vi "MGCC_FntStaMach_Control panel loop.vi"   [LabVIEW 2016]
doc: "This VI is used to convert the flags into events."
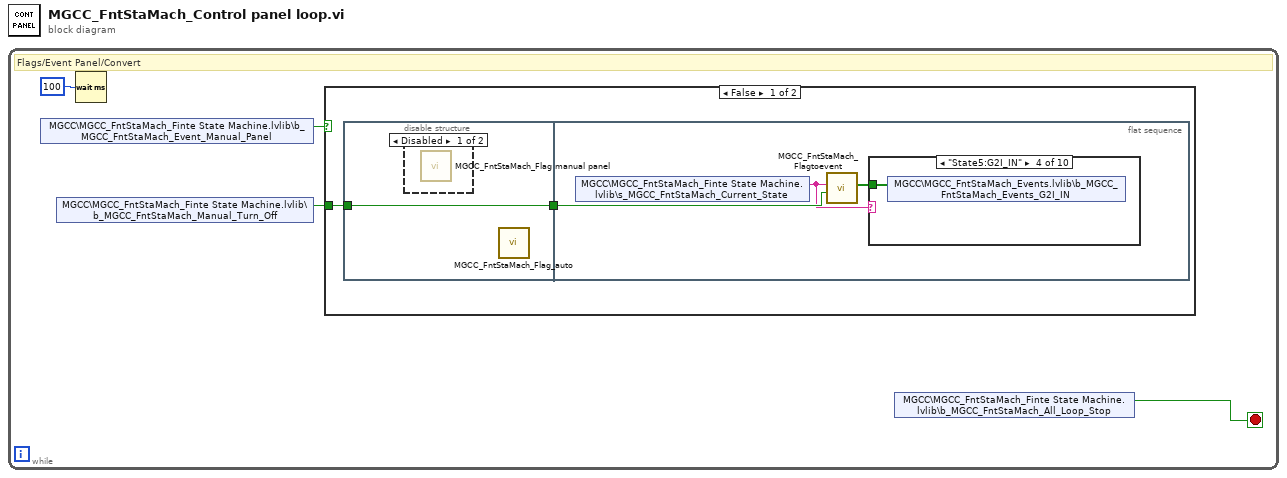
[diagram p0: block diagram]
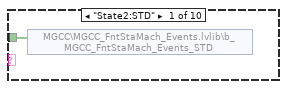
[diagram p3: hidden frame]
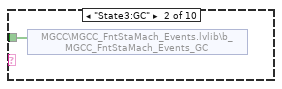
[diagram p4: hidden frame]
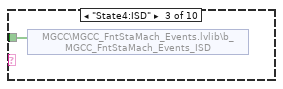
[diagram p5: hidden frame]
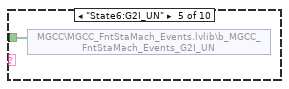
[diagram p6: hidden frame]
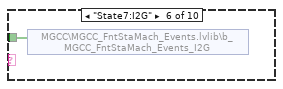
[diagram p7: hidden frame]
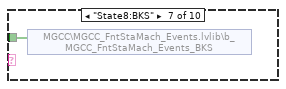
[diagram p8: hidden frame]
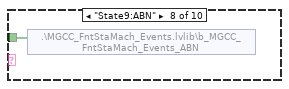
[diagram p9: hidden frame]
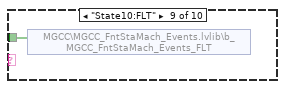
[diagram p10: hidden frame]
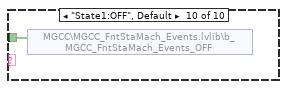
[diagram p11: hidden frame]
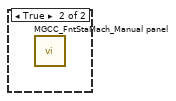
[diagram p12: hidden frame]
diagram:
  n1 = while {
    stop <- w3 stop-if-true
    # "Flags/Event Panel/Convert"
    n2 = shared-variable "MGCC\\MGCC_FntStaMach_Finte State Machine.lvlib\\b_MGCC_FntStaMach_Event_Manual_Panel"() -> (w2:bool)  [unwired: 1 in, 1 out]
    n3 = shared-variable "MGCC\\MGCC_FntStaMach_Finte State Machine.lvlib\\b_MGCC_FntStaMach_Manual_Turn_Off"() -> (w1:bool)  [unwired: 1 in, 1 out]
    n4 = Wait (ms)(milliseconds to wait=u32 100) -> ()  [unwired: 1 out]
    n5 = case shown="False" w2 {
      tunnel: w1 -> [w6 _]
      frame False {
        n6 = flat-sequence {
          tunnel: w6 -> [w7]
          tunnel: [w7] -> w5
          tunnel: w5 -> [w10]
          frame #0 {
            n7 = disable-structure shown="Disabled" {
              frame Disabled {
                n8 = call "MGCC_FntStaMach_Flag manual panel.vi"() -> ()  [unwired: 12 in]
              }
              frame Enabled {
              }
            }
            n9 = call "MGCC_FntStaMach_Flag_auto.vi"() -> ()  [unwired: 1 out]
          }
          frame #1 {
            n10 = shared-variable "MGCC\\MGCC_FntStaMach_Finte State Machine.lvlib\\s_MGCC_FntStaMach_Current_State"() -> (w8:string)  [unwired: 1 in, 1 out]
            n11 = call "MGCC_FntStaMach_Flagtoevent.vi"("M_OFF"=w10, "Pre_state"=w8) -> ("Event"=w9:bool[])  [unwired: 8 in, 1 out]
            n12 = case shown="\"State5:G2I_IN\"" w8 {
              tunnel: w9 -> [w11 w12 w13 w14 w15 w16 w17 w18 w19 w20]
              frame "State2:STD" {
                n13 = shared-variable "MGCC\\MGCC_FntStaMach_Events.lvlib\\b_MGCC_FntStaMach_Events_STD"(w11) -> ()  [unwired: 1 in, 1 out]
              }
              frame "State3:GC" {
                n14 = shared-variable "MGCC\\MGCC_FntStaMach_Events.lvlib\\b_MGCC_FntStaMach_Events_GC"(w12) -> ()  [unwired: 1 in, 1 out]
              }
              frame "State4:ISD" {
                n15 = shared-variable "MGCC\\MGCC_FntStaMach_Events.lvlib\\b_MGCC_FntStaMach_Events_ISD"(w13) -> ()  [unwired: 1 in, 1 out]
              }
              frame "State5:G2I_IN" {
                n16 = shared-variable "MGCC\\MGCC_FntStaMach_Events.lvlib\\b_MGCC_FntStaMach_Events_G2I_IN"(w14) -> ()  [unwired: 1 in, 1 out]
              }
              frame "State6:G2I_UN" {
                n17 = shared-variable "MGCC\\MGCC_FntStaMach_Events.lvlib\\b_MGCC_FntStaMach_Events_G2I_UN"(w15) -> ()  [unwired: 1 in, 1 out]
              }
              frame "State7:I2G" {
                n18 = shared-variable "MGCC\\MGCC_FntStaMach_Events.lvlib\\b_MGCC_FntStaMach_Events_I2G"(w16) -> ()  [unwired: 1 in, 1 out]
              }
              frame "State8:BKS" {
                n19 = shared-variable "MGCC\\MGCC_FntStaMach_Events.lvlib\\b_MGCC_FntStaMach_Events_BKS"(w17) -> ()  [unwired: 1 in, 1 out]
              }
              frame "State9:ABN" {
                n20 = shared-variable ".\\MGCC_FntStaMach_Events.lvlib\\b_MGCC_FntStaMach_Events_ABN"(w18) -> ()  [unwired: 1 in, 1 out]
              }
              frame "State10:FLT" {
                n21 = shared-variable "MGCC\\MGCC_FntStaMach_Events.lvlib\\b_MGCC_FntStaMach_Events_FLT"(w19) -> ()  [unwired: 1 in, 1 out]
              }
              frame "State1:OFF", Default {
                n22 = shared-variable "MGCC\\MGCC_FntStaMach_Events.lvlib\\b_MGCC_FntStaMach_Events_OFF"(w20) -> ()  [unwired: 1 in, 1 out]
              }
            }
          }
        }
      }
      frame True {
        n23 = call "MGCC_FntStaMach_Manual panel.vi"() -> ()  [unwired: 1 in, 1 out]
      }
    }
    n24 = shared-variable "MGCC\\MGCC_FntStaMach_Finte State Machine.lvlib\\b_MGCC_FntStaMach_All_Loop_Stop"() -> (w3:bool)  [unwired: 1 in, 1 out]
  }
